vi "test Set-Get Description.vi"(8 "error in":errorcluster, 11 "TestCase in":refnum<class "Scripting.lvclass">) -> (0 "error out":errorcluster, 3 "TestCase out":refnum<class "Scripting.lvclass">)   [LabVIEW 2020, in "Scripting.lvclass"]
uses:
  Scripting.lvclass
  <vilib>/addons/_JKI Toolkits/VI Tester/TestCase.llb/TestCase.lvclass
  Scripting/AIM MIL-STD-1553 Scripting.lvlib
  <vilib>/numeric/Random Number (Range) U64.vi
  C:/dev/git/niveristand-custom-device-testing-tools/VeriStandScriptingTestCase/VeriStandScriptingTestCase.lvclass
  C:/Program Files (x86)/National Instruments/LabVIEW 2020/vi.lib/addons/_JKI Toolkits/VI Tester/TestCase.llb/TestCase.lvclass
  C:/dev/git/niveristand-aim-milStd1553-custom-device/Source/Custom Device Support/Tests/Unit/Scripting/Scripting.lvclass
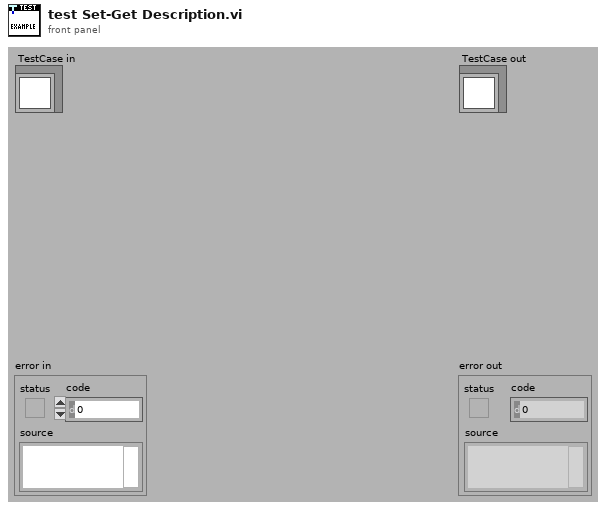
[diagram p1: front panel]
types:
  T1 = typedef "Custom Device API.lvlib/Custom Device Item Ref.ctl" = u64
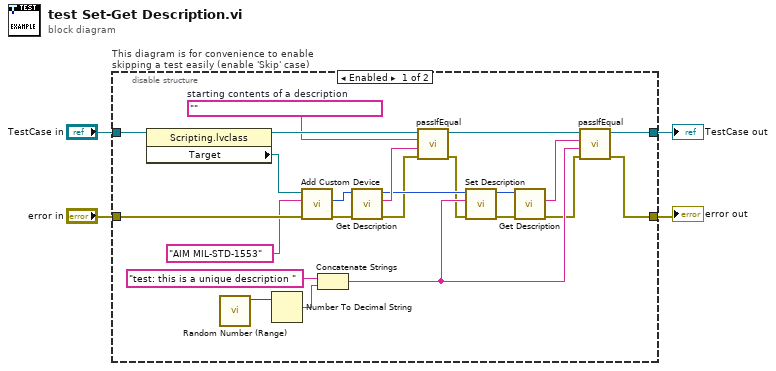
[diagram p0: block diagram]
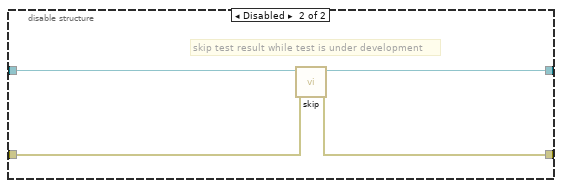
[diagram p2: hidden frame]
diagram:
  n1 = disable-structure "This diagram is for convenience to enable skipping a test easily (enable 'Skip' case)" shown="Enabled" {
    disable-tunnel: "TestCase in" -> [w23 w31]
    disable-tunnel: [w25 w29] -> w1
    disable-tunnel: [w24 w30] -> w3
    disable-tunnel: "error in" -> [w27 w28]
    frame Enabled {
      w17 = ""  # starting contents of a description
      n2 = property class="Scripting.lvclass"(reference=w23) -> (reference out=w21:refnum<class "Scripting.lvclass">, "Target"=w22:refnum<k24>)  [unwired: 1 in, 1 out]
      n3 = call-poly <vilib>:"Random Number (Range).vi"() -> ("number"=w10:u64)  [unwired: 11 in]
      n4 = Number To Decimal String(number=w10) -> (decimal integer string=w9:string)  [unwired: 1 in]
      n5 = call "Add Custom Device.vi"("error in"=w27, "custom device name"="AIM MIL-STD-1553" ("name"), "target"=w22) -> ("error out"=w20:errorcluster, "custom device"=w19:T1)  [unwired: 6 in, 1 out]
      n6 = Concatenate Strings("test: this is a unique description " ("name"), w9) -> (w8:string)
      n7 = call "Get Description.vi"("error in"=w20, "custom device"=w19) -> ("error out"=w7:errorcluster, "description"=w18:string, "custom device out"=w16:T1)  [unwired: 7 in]
      n8 = call-dynamic "passIfEqual.vi"("error in (no error)"=w7, "y"=w18, "x"=w17, "TestCase in"=w21) -> ("error out"=w6:errorcluster, "TestCase out"=w13:refnum<class "Scripting.lvclass">)  [unwired: 6 in]
      n9 = call "Set Description.vi"("error in"=w6, "description"=w8, "custom device"=w16) -> ("error out"=w15:errorcluster, "custom device out"=w14:T1)  [unwired: 7 in]
      n10 = call "Get Description.vi"("error in"=w15, "custom device"=w14) -> ("error out"=w5:errorcluster, "description"=w12:string)  [unwired: 7 in, 1 out]
      n11 = call-dynamic "passIfEqual.vi"("error in (no error)"=w5, "y"=w8, "x"=w12, "TestCase in"=w13) -> ("error out"=w24:errorcluster, "TestCase out"=w25:refnum<class "Scripting.lvclass">)  [unwired: 6 in]
    }
    frame Disabled {
      # "skip test result while test is under development"
      n12 = call <vilib>:"skip.vi"("error in (no error)"=w28, "TestCase in"=w31) -> ("error out"=w30:errorcluster, "TestCase out"=w29:refnum<class "Scripting.lvclass">)  [unwired: 8 in]
    }
  }
  "error out" <- w3
  "TestCase out" <- w1
